vi "crc32_String.vi"(0 "String in":string, 1 "CRC32 Buffer":u32 format="%.0x") -> (2 "CRC32":u32 format="%.0x")   [LabVIEW 2017, in "Test Executive Builder Model.lvclass"]
uses:
  <vilib>/gpm_packages/@cs/Test-executive-builder/Source/Test Executive Builder Model/Test Executive Builder Model/Test Executive Builder Model.lvclass
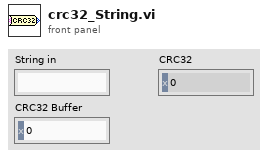
[diagram p1: front panel]
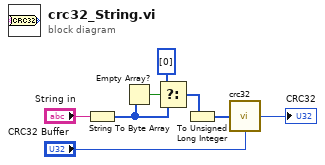
[diagram p0: block diagram]
diagram:
  n1 = String To Byte Array(string="String in") -> (unsigned byte array=w5:u8[])
  n2 = Empty Array?(array=w5) -> (empty?=w7:bool)
  n3 = Select(t=u8[] [0], s=w7, f=w5) -> (s? t:f=w4:u8[])
  n4 = To Unsigned Long Integer(number=w4) -> (unsigned 32bit integer=w3:u32[])
  n5 = call <vilib>:"crc32.vi"("Data in"=w3, "CRC32 Buffer"="CRC32 Buffer") -> ("CRC32"=→"CRC32":u32)
